vi "Main_Moving_Average_Stack.vi"(0 "Generated_Data_In":dbl, 11 "Error_In":errorcluster, 13 "Operation":T1=enum."Push") -> (4 "Generated_Data_Out":dbl, 6 "Generated_Data_Preview":dbl[](array[numeric]), 8 "Overflow":bool, 10 "Underflow":bool, 15 "Error_Out":errorcluster)   [LabVIEW 2023]
doc: "It is a Stack used to send data to other VIs or loops."
uses:
  Controls/Operation_Select_Stack.ctl
  Controls/Stack_and_Parameter.ctl
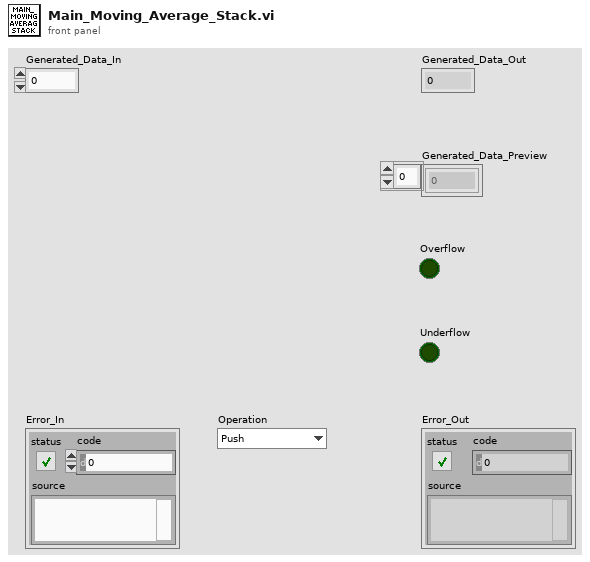
[diagram p1: front panel]
types:
  T1 = typedef "Operation_Select_Stack.ctl" = enum16{"Initialize", "Push", "Pop", "Preview"}
  T2 = typedef "Stack_and_Parameter.ctl" = cluster{"Head_Pointer":i32, "Dimention_Size":i32, "Generated_Data":dbl[]}
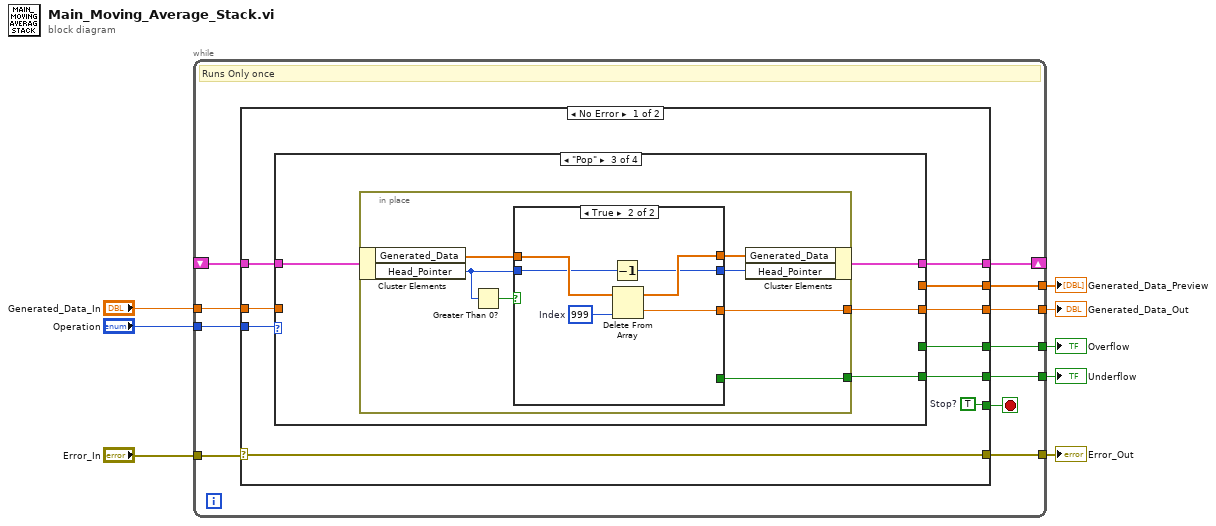
[diagram p0: block diagram]
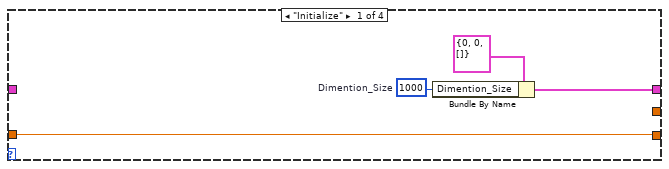
[diagram p2: hidden frame]
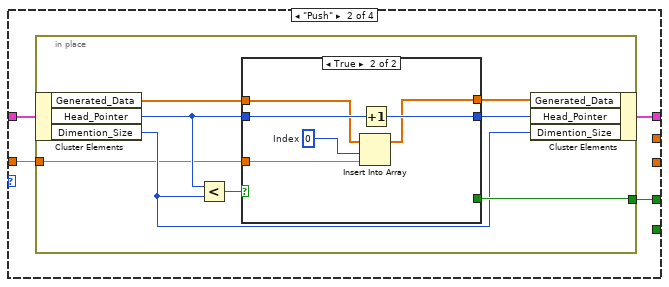
[diagram p3: hidden frame]
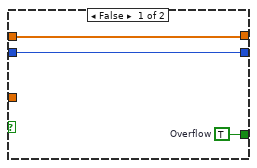
[diagram p4: hidden frame]
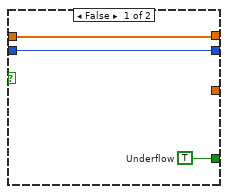
[diagram p5: hidden frame]
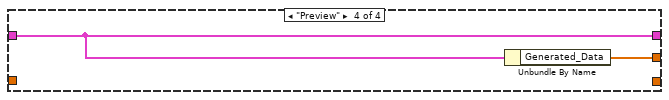
[diagram p6: hidden frame]
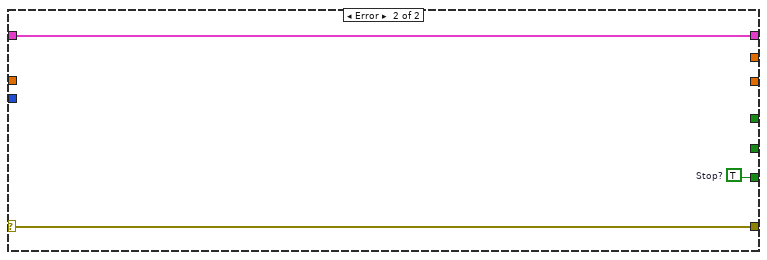
[diagram p7: hidden frame]
diagram:
  n1 = while {
    tunnel: [w19] -> w2
    tunnel: "Operation" -> [w18]
    tunnel: [w16] -> w7
    tunnel: [w15] -> w6
    shift-right: [w14] -> _
    shift-left: _ -> [w13]
    tunnel: "Error_In" -> [w12]
    tunnel: [w11] -> w4
    tunnel: "Generated_Data_In" -> [w10]
    tunnel: [w9] -> w1
    stop <- w17 stop-if-true
    # "Runs Only once"
    n2 = case shown="No Error" w12 {
      selector: w12 -> [w22 w77]
      tunnel: [w29 _] -> w19
      tunnel: w18 -> [w28 _]
      tunnel: [w27 w78] -> w17
      tunnel: [w26 _] -> w16
      tunnel: [w25 _] -> w15
      tunnel: [w24 w79] -> w14
      tunnel: w13 -> [w23 w79]
      tunnel: [w22 w77] -> w11
      tunnel: w10 -> [w21 _]
      tunnel: [w20 _] -> w9
      frame No Error {
        w27 = TRUE  # Stop?
        n3 = case shown="\"Pop\"" w28 {
          tunnel: w23 -> [_ w36 w55 w76]
          tunnel: [w30 _ w58 _] -> w29
          tunnel: [_ w37 _ _] -> w26
          tunnel: [_ _ w57 _] -> w25
          tunnel: [w33 w35 w56 w76] -> w24
          tunnel: w21 -> [w30 w34 _ _]
          tunnel: [_ _ _ w75] -> w20
          frame "Initialize" {
            w31 = 1000  # Dimention_Size
            n4 = Bundle By Name(cluster=T2 {"Head_Pointer"=0, "Dimention_Size"=0, "Generated_Data"=[]}, "Dimention_Size"=w31) -> (w33:T2)
          }
          frame "Push" {
            n5 = in-place "In Place Element Structure" {
              in-place-border: [w44] -> w37
              in-place-border: w34 -> [w38]
              n6 = in-place-cluster #1(w36) -> ("Generated_Data"=w43:dbl[], "Head_Pointer"=w40:i32, "Dimention_Size"=w39:i32)
              n7 = Less?(x=w40, y=w39) -> (x < y?=w45:bool)
              n8 = case shown="True" w45 {
                tunnel: w43 -> [w47 w51]
                tunnel: [w47 w52] -> w41
                tunnel: w40 -> [w48 w54]
                tunnel: [w48 w53] -> w42
                tunnel: [w46 _] -> w44
                tunnel: w38 -> [_ w50]
                frame False {
                  w46 = TRUE  # Overflow
                }
                frame True {
                  w49 = 0  # Index
                  n9 = Insert Into Array(array=w51, index=w49, new element=w50) -> (w52:dbl[])
                  n10 = Increment(x=w54) -> (x+1=w53:i32)
                }
              }
              n11 = in-place-cluster #1("Generated_Data"=w41, "Head_Pointer"=w42, "Dimention_Size"=w39) -> (w35:T2)
            }
          }
          frame "Pop" {
            n12 = in-place "In Place Element Structure" {
              in-place-border: [w65] -> w58
              in-place-border: [w63] -> w57
              n13 = in-place-cluster #2(w55) -> ("Generated_Data"=w60:dbl[], "Head_Pointer"=w61:i32)
              n14 = Greater Than 0?(x=w61) -> (x > 0?=w62:bool)
              n15 = case shown="True" w62 {
                tunnel: [w68 w73] -> w59
                tunnel: w60 -> [w68 w74]
                tunnel: [_ w72] -> w65
                tunnel: w61 -> [w67 w71]
                tunnel: [w67 w70] -> w64
                tunnel: [w66 _] -> w63
                frame False {
                  w66 = TRUE  # Underflow
                }
                frame True {
                  w69 = 999  # Index
                  n16 = Decrement(x=w71) -> (x-1=w70:i32)
                  n17 = Delete From Array(array=w74, index=w69) -> (deleted portion=w72:dbl, array with subset deleted=w73:dbl[])  [unwired: 1 in]
                }
              }
              n18 = in-place-cluster #2("Generated_Data"=w59, "Head_Pointer"=w64) -> (w56:T2)
            }
          }
          frame "Preview" {
            n19 = Unbundle By Name(w76) -> ("Generated_Data"=w75:dbl[])
          }
        }
      }
      frame Error {
        w78 = TRUE  # Stop?
      }
    }
  }
  "Error_Out" <- w4
  "Overflow" <- w7
  "Underflow" <- w6
  "Generated_Data_Out" <- w2
  "Generated_Data_Preview" <- w1
